vi "Judge Frame Code Exist.vi"(8 "error in (no error)":errorcluster, 10 "Online_Table.SN":string, 11 "2DA_Str":string[][](array[string])) -> (0 "error out":errorcluster, 2 "Status":bool, 3 "Frame Code":string)   [LabVIEW 2014]
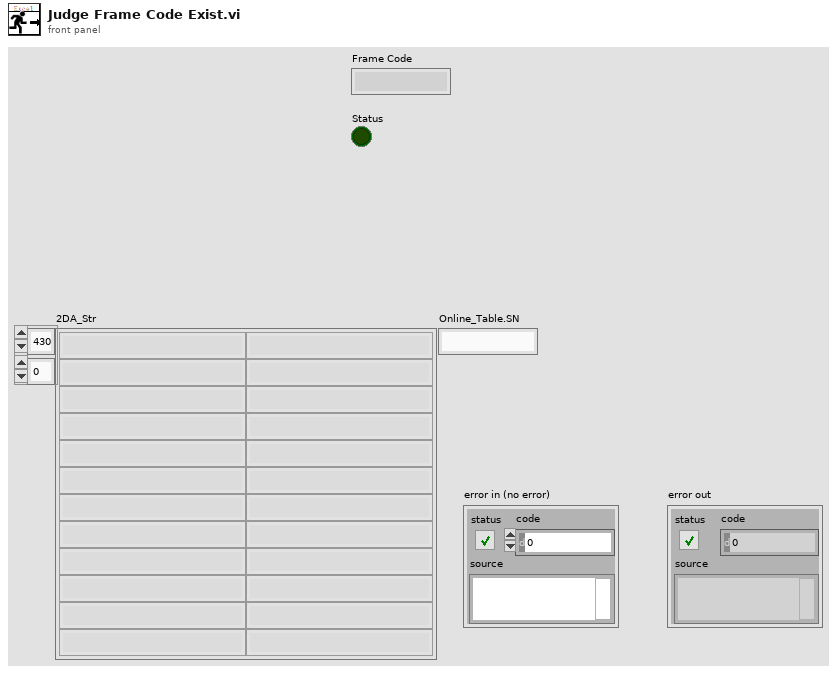
[diagram p1: front panel]
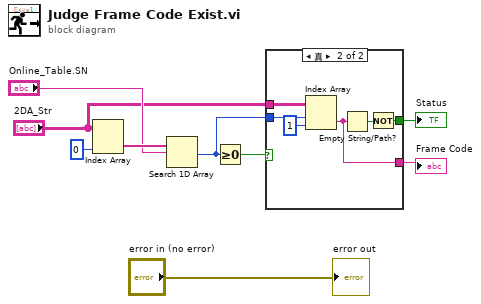
[diagram p0: block diagram]
diagram:
  n1 = Index Array(array="2DA_Str", index (col)=0 ("disabled index (col)")) -> (element=w8:string[])  [unwired: 1 in]
  n2 = Search 1D Array(1D array=w8, element="Online_Table.SN") -> (index of element=w4:i32)  [unwired: 1 in]
  n3 = Greater Or Equal To 0?(x=w4) -> (x >= 0?=w5:bool)
  n4 = case shown="真" w5 {
    tunnel: "2DA_Str" -> [_ w15]
    tunnel: w4 -> [_ w14]
    tunnel: [_ w11] -> w3
    tunnel: [_ w10] -> w1
    frame False {
    }
    frame True {
      n5 = Index Array(array=w15, index (row)=w14, index (col)=1 ("disabled index (col)")) -> (element=w10:string)
      n6 = Empty String/Path?(string/path=w10) -> (empty?=w12:bool)
      n7 = Not(x=w12) -> (.not. x?=w11:bool)
    }
  }
  "Status" <- w3
  "Frame Code" <- w1
  "error out" <- "error in (no error)"
